vi "Autonomous Independent.vi"() -> ()   [LabVIEW 2016]
doc: "This VI is called when autonomous begins, and will automatically be terminated when autonomous ends. You can carry out timed or sensor driven robot movement independently without needing to return to the caller."
uses:
  Systems/Global 1.vi
  Global 2.vi
  <vilib>/Rock Robotics/Network Tables/NT Read Number.vi
panel:
  out "Present (s)":dbl=3575828146.202245
  out "Time has Elapsed":bool=TRUE
  out "Elapsed Time (s)":dbl=0.5143580436706543
  out "Gyro":dbl=31.8801500557848
  in  "Oscillate effort":dbl=0.25 format="%#_13g"
  out "Auto Mode":dbl=5.0
  in  "Auton_Modes":T1(array[cluster])=[{"Actions"=[{"Effort"=0.55, "Duration"=3.5, "Action"=enum."Vision Correction", "Encoder"=0.0, "Condition"=FALSE}, {"Effort"=0.0, "Duration"=0.0, "Action"=enum."Nothing", "Encoder"=0.0, "Condition"=FALSE}]}, {"Actions"=[{"Effort"=0.0, "Duration"=0.1, "Action"=enum."Drive Encoder Reset", "Encoder"=0.0, "Condition"=FALSE}, {"Effort"=0.0, "Duration"=0.1, "Action"=enum."Gyro Reset", "Encoder"=0.0, "Condition"=FALSE}, {"Effort"=0.4, "Duration"=4.0, "Action"=enum."Drive", "Encoder"=62.0, "Condition"=FALSE}, {"Effort"=0.18, "Duration"=1.0, "Action"=enum."Turn", "Encoder"=-60.0, "Condition"=FALSE}, {"Effort"=0.0, "Duration"=0.1, "Action"=enum."Drive Encoder Reset", "Encoder"=0.0, "Condition"=FALSE}, {"Effort"=0.4, "Duration"=4.0, "Action"=enum."Drive", "Encoder"=65.5, "Condition"=FALSE}, {"Effort"=1.0, "Duration"=0.25, "Action"=enum."Gear0", "Encoder"=0.0, "Condition"=FALSE}, {"Effort"=-0.3, "Duration"=0.1, "Action"=enum."Drive Encoder Reset", "Encoder"=24.0, "Condition"=FALSE}, {"Effort"=-0.4, "Duration"=3.0, "Action"=enum."Drive", "Encoder"=36.0, "Condition"=FALSE}, {"Effort"=0.0, "Duration"=0.0, "Action"=enum."Turn", "Encoder"=31.5, "Condition"=FALSE}, {"Effort"=0.0, "Duration"=0.1, "Action"=enum."Drive Encoder Reset", "Encoder"=0.0, "Condition"=FALSE}, {"Effort"=-0.4, "Duration"=5.0, "Action"=enum."Drive", "Encoder"=70.0, "Condition"=TRUE}]}, {"Actions"=[{"Effort"=0.0, "Duration"=0.1, "Action"=enum."Drive Encoder Reset", "Encoder"=0.0, "Condition"=FALSE}, {"Effort"=0.0, "Duration"=0.1, "Action"=enum."Gyro Reset", "Encoder"=0.0, "Condition"=FALSE}, {"Effort"=0.3, "Duration"=4.0, "Action"=enum."Drive", "Encoder"=75.0, "Condition"=FALSE}, {"Effort"=1.0, "Duration"=1.0, "Action"=enum."Gear0", "Encoder"=0.0, "Condition"=FALSE}, {"Effort"=1.0, "Duration"=0.0, "Action"=enum."Nothing", "Encoder"=0.0, "Condition"=FALSE}, {"Effort"=1.0, "Duration"=0.0, "Action"=enum."Nothing", "Encoder"=0.0, "Condition"=FALSE}, {"Effort"=0.0, "Duration"=0.0, "Action"=enum."Drive Encoder Reset", "Encoder"=0.0, "Condition"=FALSE}, {"Effort"=0.0, "Duration"=0.0, "Action"=enum."Nothing", "Encoder"=0.0, "Condition"=FALSE}, {"Effort"=0.0, "Duration"=0.0, "Action"=enum."Nothing", "Encoder"=0.0, "Condition"=FALSE}, {"Effort"=-0.2, "Duration"=10000.0, "Action"=enum."Drive", "Encoder"=24.0, "Condition"=FALSE}, {"Effort"=0.0, "Duration"=0.0, "Action"=enum."Drive Encoder Reset", "Encoder"=0.0, "Condition"=FALSE}, {"Effort"=-0.4, "Duration"=5.0, "Action"=enum."Nothing", "Encoder"=70.0, "Condition"=FALSE}]}, {"Actions"=[{"Effort"=0.0, "Duration"=0.1, "Action"=enum."Drive Encoder Reset", "Encoder"=6.462, "Condition"=FALSE}, {"Effort"=0.0, "Duration"=0.1, "Action"=enum."Gyro Reset", "Encoder"=0.0, "Condition"=FALSE}, {"Effort"=-0.25, "Duration"=1.0, "Action"=enum."Drive", "Encoder"=6.462, "Condition"=FALSE}, {"Effort"=0.0, "Duration"=0.1, "Action"=enum."Gyro Reset", "Encoder"=0.0, "Condition"=FALSE}, {"Effort"=-0.25, "Duration"=0.0, "Action"=enum."Turn", "Encoder"=0.0, "Condition"=FALSE}, {"Effort"=-0.25, "Duration"=0.0, "Action"=enum."Drive", "Encoder"=7.5, "Condition"=FALSE}, {"Effort"=-1.0, "Duration"=0.0, "Action"=enum."Gear0", "Encoder"=0.0, "Condition"=FALSE}, {"Effort"=0.25, "Duration"=0.0, "Action"=enum."Drive", "Encoder"=3.0, "Condition"=FALSE}]}, {"Actions"=[{"Effort"=0.0, "Duration"=0.1, "Action"=enum."Drive Encoder Reset", "Encoder"=6.462, "Condition"=FALSE}, {"Effort"=0.0, "Duration"=0.1, "Action"=enum."Gyro Reset", "Encoder"=0.0, "Condition"=FALSE}, {"Effort"=-0.25, "Duration"=1.0, "Action"=enum."Drive", "Encoder"=6.462, "Condition"=FALSE}, {"Effort"=0.0, "Duration"=0.1, "Action"=enum."Gyro Reset", "Encoder"=0.0, "Condition"=FALSE}, {"Effort"=-0.25, "Duration"=0.0, "Action"=enum."Turn", "Encoder"=0.0, "Condition"=FALSE}, {"Effort"=-0.25, "Duration"=0.0, "Action"=enum."Drive", "Encoder"=7.5, "Condition"=FALSE}, {"Effort"=-1.0, "Duration"=0.0, "Action"=enum."Gear0", "Encoder"=0.0, "Condition"=FALSE}, {"Effort"=0.25, "Duration"=0.0, "Action"=enum."Drive", "Encoder"=3.0, "Condition"=FALSE}]}, {"Actions"=[{"Effort"=0.0, "Duration"=0.1, "Action"=enum."Drive Encoder Reset", "Encoder"=0.0, "Condition"=FALSE}, {"Effort"=0.0, "Duration"=0.1, "Action"=enum."Gyro Reset", "Encoder"=0.0, "Condition"=FALSE}, {"Effort"=0.4, "Duration"=4.0, "Action"=enum."Drive", "Encoder"=62.0, "Condition"=FALSE}, {"Effort"=0.18, "Duration"=0.1, "Action"=enum."Turn", "Encoder"=60.0, "Condition"=FALSE}, {"Effort"=0.0, "Duration"=0.1, "Action"=enum."Drive Encoder Reset", "Encoder"=0.0, "Condition"=FALSE}, {"Effort"=0.4, "Duration"=4.0, "Action"=enum."Drive", "Encoder"=65.5, "Condition"=FALSE}, {"Effort"=1.0, "Duration"=0.25, "Action"=enum."Gear0", "Encoder"=0.0, "Condition"=FALSE}, {"Effort"=0.0, "Duration"=0.1, "Action"=enum."Drive Encoder Reset", "Encoder"=3.0, "Condition"=FALSE}, {"Effort"=-0.4, "Duration"=3.0, "Action"=enum."Drive", "Encoder"=36.0, "Condition"=FALSE}, {"Effort"=0.0, "Duration"=0.0, "Action"=enum."Turn", "Encoder"=31.5, "Condition"=FALSE}, {"Effort"=0.0, "Duration"=0.1, "Action"=enum."Drive Encoder Reset", "Encoder"=0.0, "Condition"=FALSE}, {"Effort"=-0.4, "Duration"=5.0, "Action"=enum."Drive", "Encoder"=70.0, "Condition"=TRUE}]}, {"Actions"=[{"Effort"=0.0, "Duration"=0.1, "Action"=enum."Nothing", "Encoder"=0.0, "Condition"=FALSE}, {"Effort"=0.0, "Duration"=0.1, "Action"=enum."Gyro Reset", "Encoder"=0.0, "Condition"=FALSE}, {"Effort"=0.25, "Duration"=5.0, "Action"=enum."Drive", "Encoder"=60000.0, "Condition"=TRUE}, {"Effort"=0.75, "Duration"=1.0, "Action"=enum."Nothing", "Encoder"=0.0, "Condition"=FALSE}, {"Effort"=0.0, "Duration"=1.0, "Action"=enum."Nothing", "Encoder"=0.0, "Condition"=FALSE}, {"Effort"=0.0, "Duration"=0.0, "Action"=enum."Nothing", "Encoder"=0.0, "Condition"=FALSE}]}, {"Actions"=[{"Effort"=0.0, "Duration"=0.1, "Action"=enum."Drive Encoder Reset", "Encoder"=0.0, "Condition"=FALSE}, {"Effort"=0.0, "Duration"=0.1, "Action"=enum."Gyro Reset", "Encoder"=0.0, "Condition"=FALSE}, {"Effort"=0.3, "Duration"=0.0, "Action"=enum."Drive", "Encoder"=24.0, "Condition"=FALSE}, {"Effort"=0.3, "Duration"=3.0, "Action"=enum."Nothing", "Encoder"=0.0, "Condition"=FALSE}, {"Effort"=0.3, "Duration"=2.0, "Action"=enum."Vision Correction", "Encoder"=30.0, "Condition"=FALSE}, {"Effort"=0.2, "Duration"=1.0, "Action"=enum."Drive", "Encoder"=18.5, "Condition"=TRUE}, {"Effort"=1.0, "Duration"=0.0, "Action"=enum."Gear0", "Encoder"=0.0, "Condition"=FALSE}, {"Effort"=-0.2, "Duration"=1.3, "Action"=enum."Drive", "Encoder"=30.0, "Condition"=TRUE}, {"Effort"=0.0, "Duration"=3.0, "Action"=enum."Nothing", "Encoder"=0.0, "Condition"=FALSE}, {"Effort"=0.03, "Duration"=0.0, "Action"=enum."Turn", "Encoder"=0.0, "Condition"=FALSE}, {"Effort"=0.0, "Duration"=0.0, "Action"=enum."Drive", "Encoder"=0.0, "Condition"=FALSE}]}, {"Actions"=[{"Effort"=0.0, "Duration"=0.0, "Action"=enum."Nothing", "Encoder"=0.0, "Condition"=FALSE}]}, {"Actions"=[{"Effort"=0.0, "Duration"=2.5, "Action"=enum."Shoot", "Encoder"=0.0, "Condition"=FALSE}, {"Effort"=0.0, "Duration"=5.0, "Action"=enum."Index", "Encoder"=0.0, "Condition"=FALSE}, {"Effort"=0.25, "Duration"=3.5, "Action"=enum."Nothing", "Encoder"=88.0, "Condition"=FALSE}, {"Effort"=1.0, "Duration"=1.0, "Action"=enum."Nothing", "Encoder"=0.0, "Condition"=FALSE}, {"Effort"=1.0, "Duration"=1.0, "Action"=enum."Nothing", "Encoder"=0.0, "Condition"=FALSE}, {"Effort"=1.0, "Duration"=0.5, "Action"=enum."Nothing", "Encoder"=0.0, "Condition"=FALSE}, {"Effort"=0.0, "Duration"=0.0, "Action"=enum."Nothing", "Encoder"=0.0, "Condition"=FALSE}, {"Effort"=-0.25, "Duration"=0.0, "Action"=enum."Nothing", "Encoder"=3.0, "Condition"=FALSE}, {"Effort"=0.0, "Duration"=0.0, "Action"=enum."Nothing", "Encoder"=0.0, "Condition"=FALSE}, {"Effort"=0.25, "Duration"=0.0, "Action"=enum."Nothing", "Encoder"=24.0, "Condition"=FALSE}, {"Effort"=0.0, "Duration"=0.0, "Action"=enum."Nothing", "Encoder"=0.0, "Condition"=FALSE}, {"Effort"=-0.25, "Duration"=0.0, "Action"=enum."Nothing", "Encoder"=12.0, "Condition"=FALSE}]}, {"Actions"=[{"Effort"=0.0, "Duration"=0.1, "Action"=enum."Drive Encoder Reset", "Encoder"=0.0, "Condition"=FALSE}, {"Effort"=0.0, "Duration"=1.0, "Action"=enum."Gyro Reset", "Encoder"=0.0, "Condition"=FALSE}, {"Effort"=0.3, "Duration"=1.4, "Action"=enum."Drive", "Encoder"=88.0, "Condition"=FALSE}, {"Effort"=0.3, "Duration"=3.0, "Action"=enum."Turn", "Encoder"=2.0, "Condition"=FALSE}, {"Effort"=1.0, "Duration"=1.0, "Action"=enum."Nothing", "Encoder"=0.0, "Condition"=FALSE}, {"Effort"=1.0, "Duration"=1.0, "Action"=enum."Nothing", "Encoder"=0.0, "Condition"=FALSE}, {"Effort"=0.0, "Duration"=0.0, "Action"=enum."Nothing", "Encoder"=0.0, "Condition"=FALSE}, {"Effort"=-0.25, "Duration"=0.0, "Action"=enum."Nothing", "Encoder"=3.0, "Condition"=FALSE}, {"Effort"=0.0, "Duration"=0.0, "Action"=enum."Nothing", "Encoder"=0.0, "Condition"=FALSE}, {"Effort"=0.25, "Duration"=0.0, "Action"=enum."Nothing", "Encoder"=24.0, "Condition"=FALSE}, {"Effort"=0.0, "Duration"=0.0, "Action"=enum."Nothing", "Encoder"=0.0, "Condition"=FALSE}, {"Effort"=-0.25, "Duration"=0.0, "Action"=enum."Nothing", "Encoder"=12.0, "Condition"=FALSE}]}, {"Actions"=[{"Effort"=0.0, "Duration"=1.0, "Action"=enum."Drive Encoder Reset", "Encoder"=0.0, "Condition"=FALSE}, {"Effort"=0.0, "Duration"=1.0, "Action"=enum."Shoot", "Encoder"=0.0, "Condition"=FALSE}, {"Effort"=0.25, "Duration"=5.0, "Action"=enum."Index", "Encoder"=88.0, "Condition"=FALSE}, {"Effort"=1.0, "Duration"=1.0, "Action"=enum."Nothing", "Encoder"=0.0, "Condition"=FALSE}, {"Effort"=1.0, "Duration"=1.0, "Action"=enum."Nothing", "Encoder"=0.0, "Condition"=FALSE}, {"Effort"=1.0, "Duration"=0.5, "Action"=enum."Nothing", "Encoder"=0.0, "Condition"=FALSE}, {"Effort"=0.0, "Duration"=0.0, "Action"=enum."Nothing", "Encoder"=0.0, "Condition"=FALSE}, {"Effort"=-0.25, "Duration"=0.0, "Action"=enum."Nothing", "Encoder"=3.0, "Condition"=FALSE}, {"Effort"=0.0, "Duration"=0.0, "Action"=enum."Nothing", "Encoder"=0.0, "Condition"=FALSE}, {"Effort"=0.25, "Duration"=0.0, "Action"=enum."Nothing", "Encoder"=24.0, "Condition"=FALSE}, {"Effort"=0.0, "Duration"=0.0, "Action"=enum."Nothing", "Encoder"=0.0, "Condition"=FALSE}, {"Effort"=-0.25, "Duration"=0.0, "Action"=enum."Nothing", "Encoder"=12.0, "Condition"=FALSE}]}, {"Actions"=[{"Effort"=0.0, "Duration"=0.1, "Action"=enum."Drive Encoder Reset", "Encoder"=0.0, "Condition"=FALSE}, {"Effort"=0.0, "Duration"=1.0, "Action"=enum."Gyro Reset", "Encoder"=0.0, "Condition"=FALSE}, {"Effort"=0.3, "Duration"=1.4, "Action"=enum."Drive", "Encoder"=88.0, "Condition"=FALSE}, {"Effort"=0.3, "Duration"=4.0, "Action"=enum."Turn", "Encoder"=0.0, "Condition"=FALSE}, {"Effort"=1.0, "Duration"=1.0, "Action"=enum."Nothing", "Encoder"=0.0, "Condition"=FALSE}, {"Effort"=1.0, "Duration"=0.5, "Action"=enum."Nothing", "Encoder"=0.0, "Condition"=FALSE}, {"Effort"=0.0, "Duration"=0.0, "Action"=enum."Nothing", "Encoder"=0.0, "Condition"=FALSE}, {"Effort"=0.3, "Duration"=0.5, "Action"=enum."Nothing", "Encoder"=24.0, "Condition"=TRUE}, {"Effort"=0.0, "Duration"=0.0, "Action"=enum."Nothing", "Encoder"=0.0, "Condition"=FALSE}, {"Effort"=-0.2, "Duration"=2.0, "Action"=enum."Nothing", "Encoder"=24.0, "Condition"=TRUE}, {"Effort"=0.0, "Duration"=0.0, "Action"=enum."Nothing", "Encoder"=0.0, "Condition"=FALSE}, {"Effort"=-0.25, "Duration"=0.0, "Action"=enum."Nothing", "Encoder"=12.0, "Condition"=FALSE}]}]
  # "Nothing"
  # "Boiler Right Right side gear"
  # "Middle Gear"
  # "Boiler Right Left Side Gear"
  # "Boiler Left RightSide Gear"
  # "Boiler Left Left Side Gear"
  # "Drive"
  # "Vision Correction"
  # "Hopper"
  # "10 ball"
  # "Farside"
  # "Boilerside-10 ball"
  # "Auto 5"
  # "Auto 6"
  # "Auto 6"
  # "Auto 7"
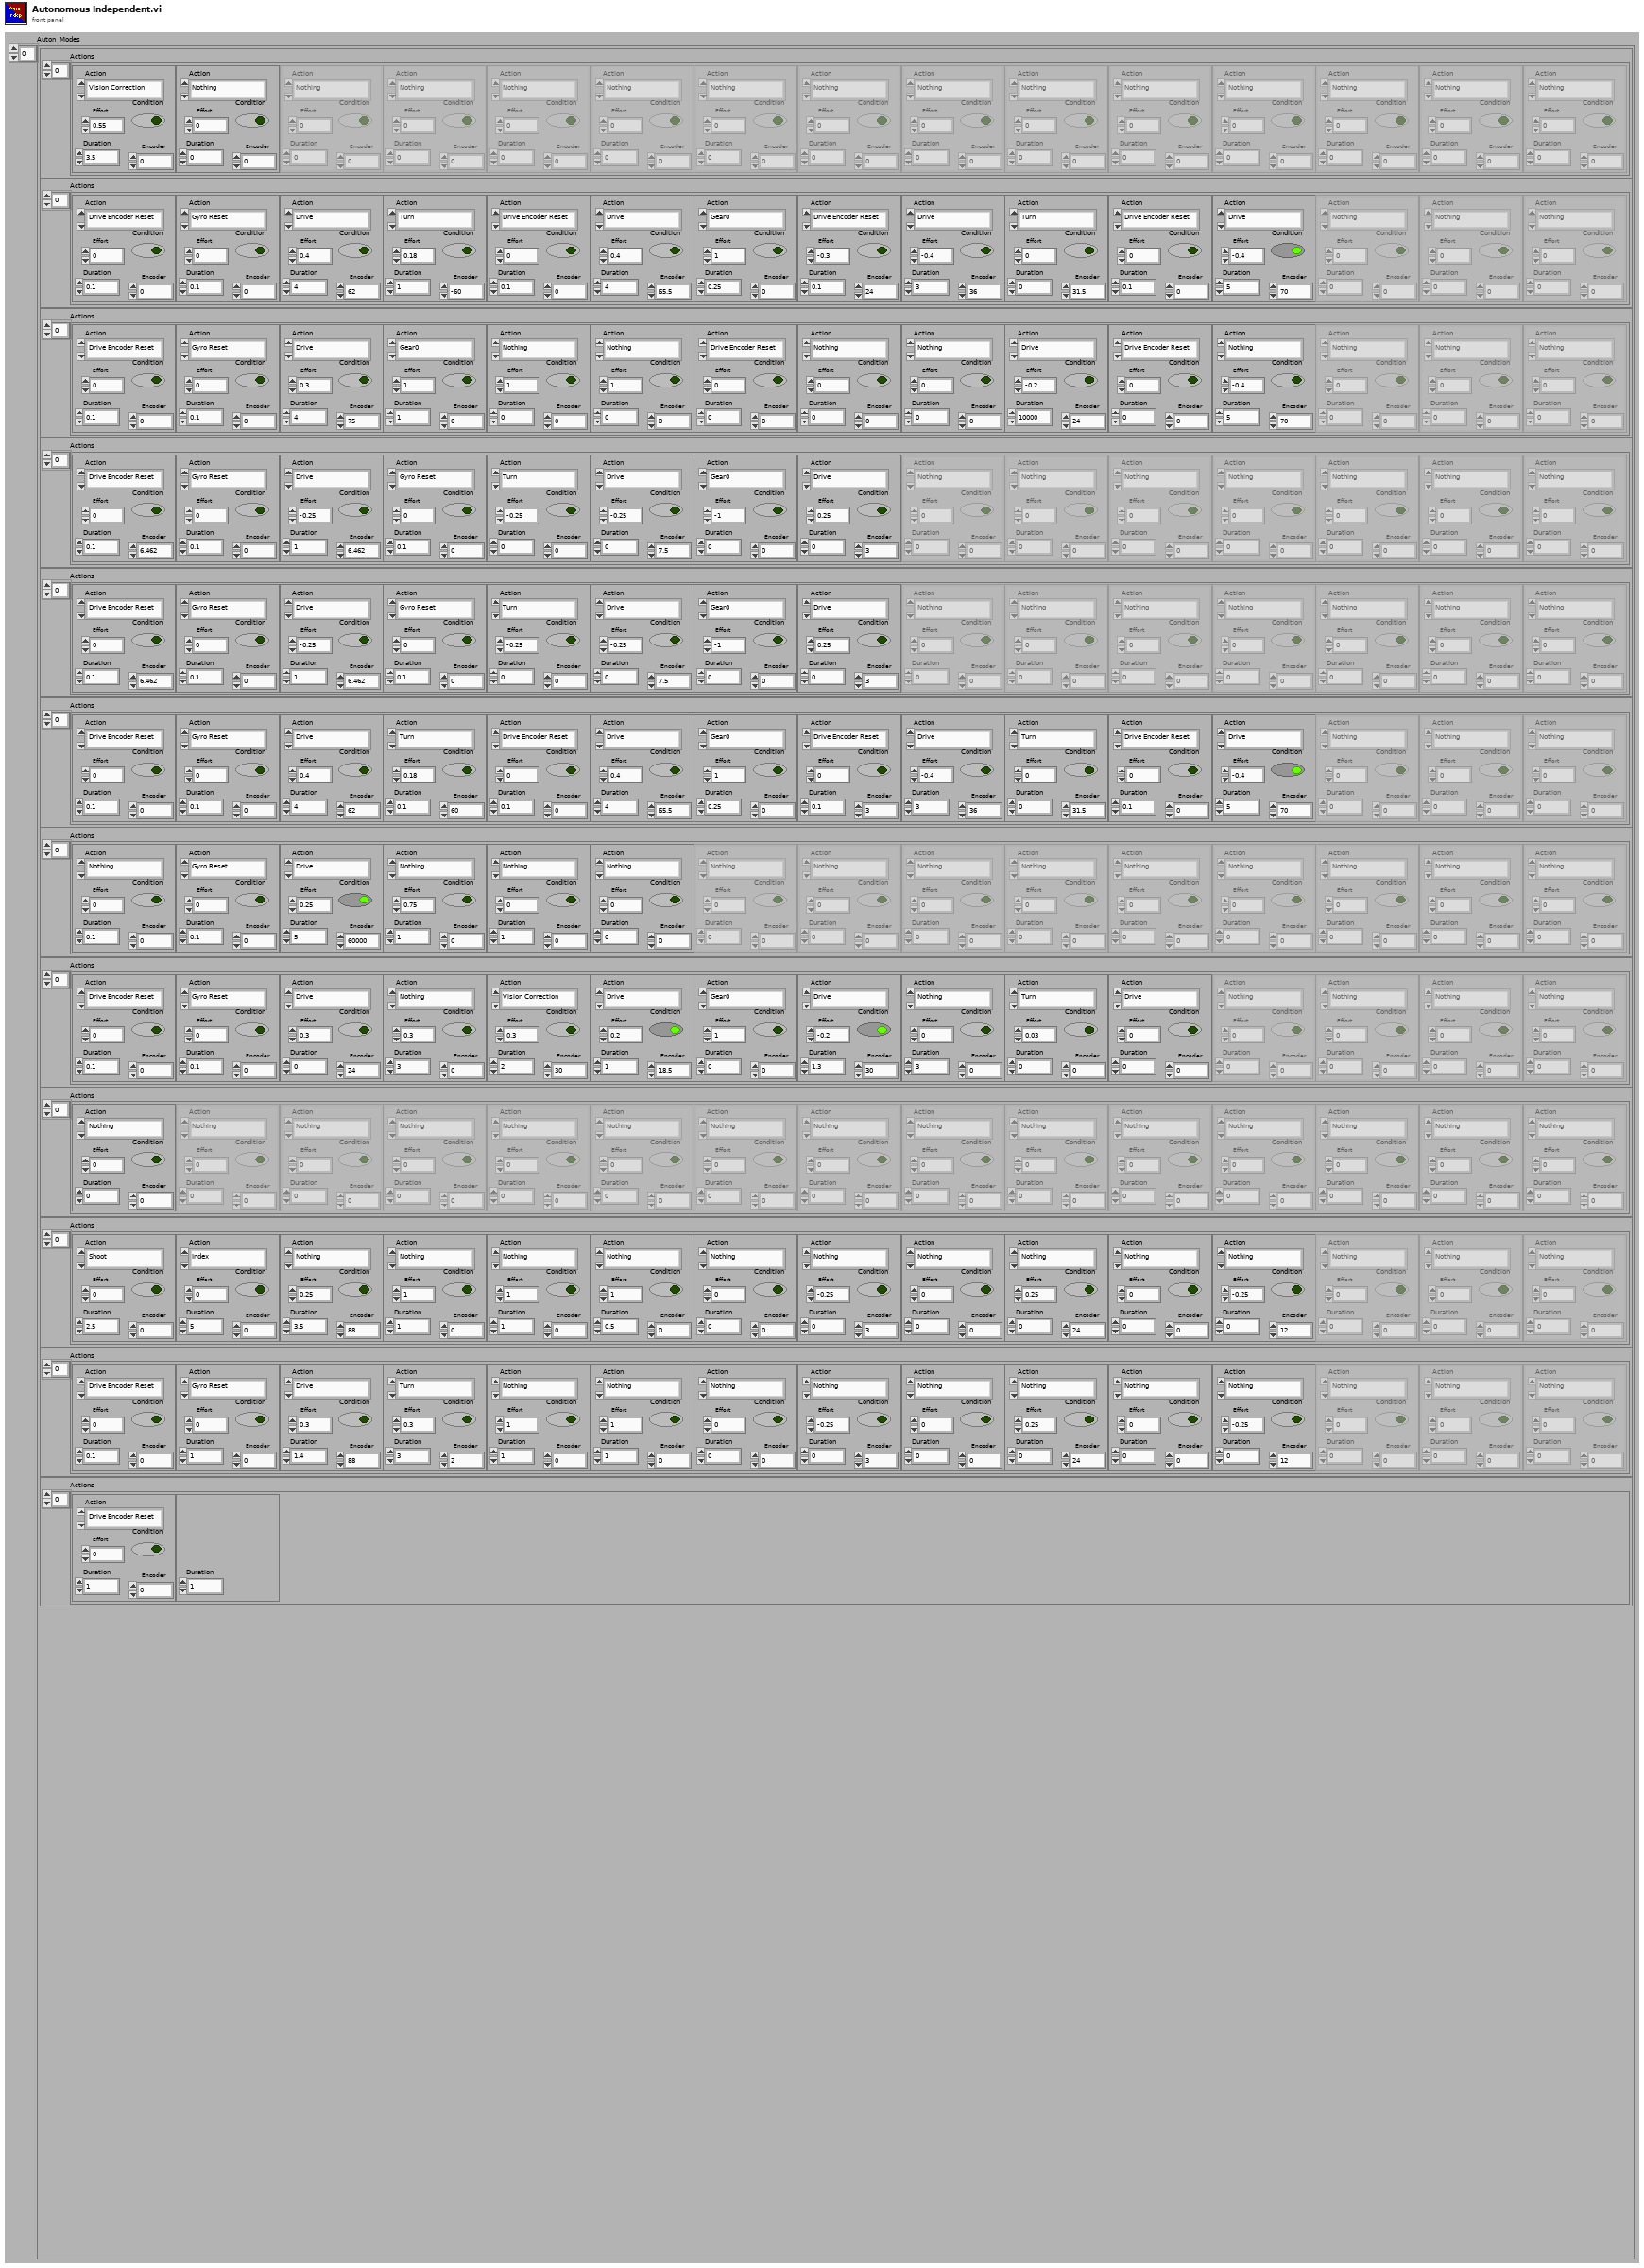
[diagram p1: front panel]
types:
  T1 = cluster{"Actions":cluster{"Effort":dbl, "Duration":dbl, "Action":enum16{"Nothing", "Drive", "Vision Correction", "Turn", "Gear0", "Gear1", "Climb", "Intake", "Index", "Shoot", "Test", "Drive Encoder Reset", "Gyro Reset"}, "Encoder":dbl, "Condition":bool}[]}[]
  T2 = cluster{"Actions":cluster{"Effort":dbl, "Duration":dbl, "Action":enum16{"Nothing", "Drive", "Vision Correction", "Turn", "Gear0", "Gear1", "Climb", "Intake", "Index", "Shoot", "Test", "Drive Encoder Reset", "Gyro Reset"}, "Encoder":dbl, "Condition":bool}[]}
  T3 = cluster{"Effort":dbl, "Duration":dbl, "Action":enum16{"Nothing", "Drive", "Vision Correction", "Turn", "Gear0", "Gear1", "Climb", "Intake", "Index", "Shoot", "Test", "Drive Encoder Reset", "Gyro Reset"}, "Encoder":dbl, "Condition":bool}[]
  T4 = enum16{"Nothing", "Drive", "Vision Correction", "Turn", "Gear0", "Gear1", "Climb", "Intake", "Index", "Shoot", "Test", "Drive Encoder Reset", "Gyro Reset"}
  T5 = typedef "WPI_MotorControlDeviceRef.ctl" = cluster{"DeviceStatus":errorcluster, "Type":T6, "PWM":cluster{"PWM Channel":T7, "DeadBand":T8}, "CAN":cluster{"Device Number":u8, "SetOutput VI Ref":variant, "GetOutput VI Ref":variant, "Enable VI Ref":variant, "Disable VI Ref":variant, "Data":variant}, "Invert":bool}
  T6 = typedef "WPI_MotorControlType.ctl" = enum16{"PWM", "CAN"}
  T7 = typedef "FPGA_DIOPWMChannel.ctl" = enum8{"PWM 0", "PWM 1", "PWM 2", "PWM 3", "PWM 4", "PWM 5", "PWM 6", "PWM 7", "PWM 8", "PWM 9", "PWM MXP 0", "PWM MXP 1", "PWM MXP 2", "PWM MXP 3", "PWM MXP 4", "PWM MXP 5", "PWM MXP 6", "PWM MXP 7", "PWM MXP 8", "PWM MXP 9", "Invalid"}
  T8 = typedef "WPI_PWMDeadband.ctl" = cluster{"Name":string, "maxPositivePwm":i32, "minPositivePwm":i32, "centerPwm":i32, "maxNegativePwm":i32, "minNegativePwm":i32, "angularRange":u16}
  T9 = typedef "WPI_CANTalonSRX_GlobalStatus.ctl" = cluster{"Applied Throttle":dbl, "Module Enabled":bool, "CAN Error":errorcluster, "Closed Loop Error":dbl, "Forward Limit Switch Closed":bool, "Reverse Limit Switch Closed":bool, "Sensor Position":dbl, "Sensor Velocity":dbl, "Current":dbl, "Sticky Fault - Over Temp":bool, "Sticky Fault - Under Voltage":bool, "Sticky Fault - Forward Limit":bool, "Sticky Fault - Reverse Limit":bool, "Sticky Fault - Forward Soft Limit":bool, "Sticky Fault - Reverse Soft Limit":bool, "Brake is Enabled":bool, "Encoder Position":dbl, "Encoder Velocity":dbl, "Encoder Index Count":dbl, "Encoder A Pin State":bool, "Encoder B Pin State":bool, "Encoder Index Pin State":bool, "Analog In":dbl, "Analog In Velocity":dbl, "Temperature (C)":dbl, "Battery Voltage":dbl, "Control 5 Is Supported":bool, "Current Profile Slot Select":dbl, "Pos Div 8":bool, "Vel Div 4":bool, "Pulse Width Position":i32, "Pulse Width Velocity":i32, "Pulse Width Rise To Rise (us)":i32, "Pulse Width Rise To Fall (us)":i32, "Mot Prof Active Is Under Run":bool, "Mot Prof Active Has Under Run":bool, "Mot Prof Active Is Last":bool, "Mot Prof Active Velocity Only":bool, "Mot Prof Active Is Valid":bool, "Mot Prof Buffer Is Full":bool, "Mot Prof Active Profile Slot Select":i32, "Mot Prof NextID":i32, "Mot Prof Count":i32, "Mot Prof Active Velocity":dbl, "Mot Prof Active Position":dbl, "Mot Prof Output Enable":i32}
  T10 = typedef "WPI_GyroDevRef.ctl" = cluster{"DevStatus":errorcluster, "Analog Channel":T11, "Offset":dbl, "Gain (VoltsPerDegree/Second)":dbl, "Gyro Type":enum16{"Analog", "XRS450"}, "Handle":i32, "SPI Bus":T12, "Device Found":bool, "Sample Rate":dbl, "Calibrate On Open":bool}
  T11 = typedef "FPGA_AIChannel.ctl" = enum8{"AI 0", "AI 1", "AI 2", "AI 3", "AI MXP 0", "AI MXP 1", "AI MXP 2", "AI MXP 3", "Invalid"}
  T12 = typedef "spi_bus.ctl" = enum16{"SPI On-Board, CS0", "SPI On-Board, CS1", "SPI On-Board, CS2", "SPI On-Board, CS3", "SPI MXP", "Invalid"}
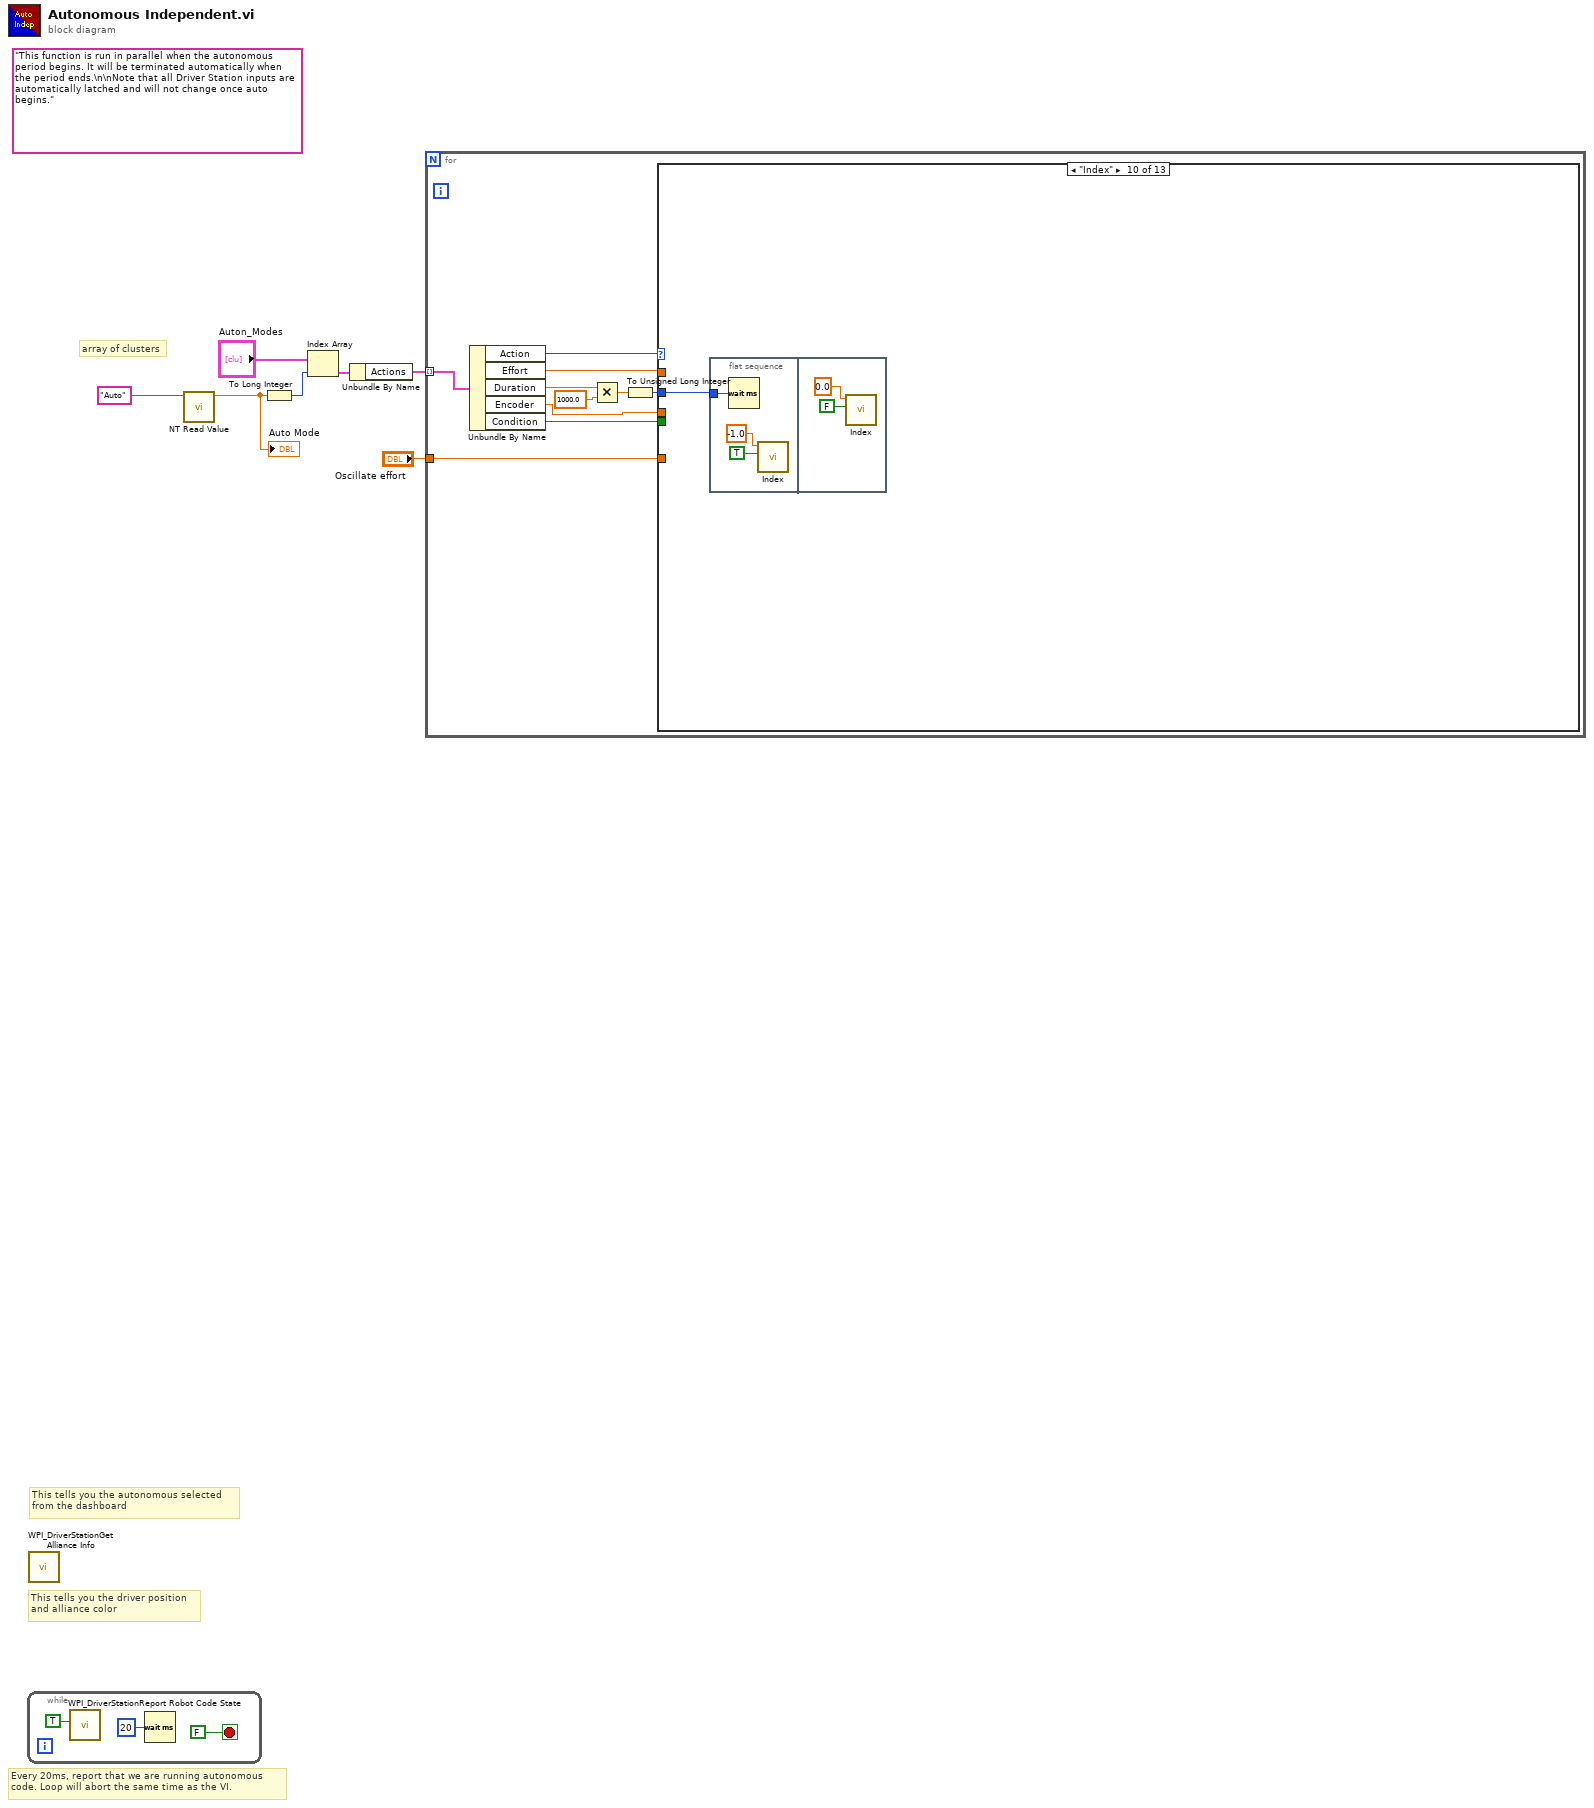
[diagram p0: block diagram]
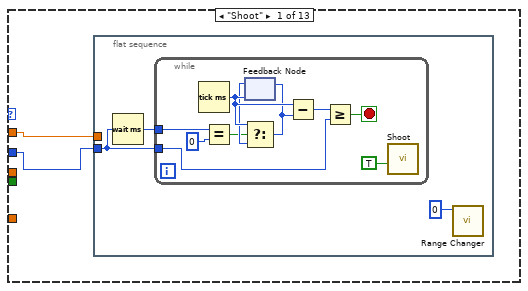
[diagram p2: hidden frame]
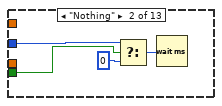
[diagram p3: hidden frame]
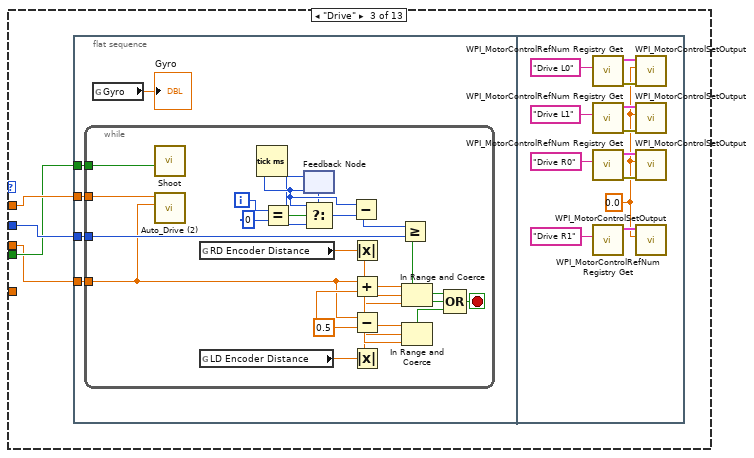
[diagram p4: hidden frame]
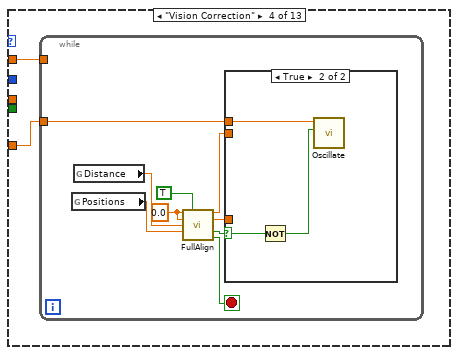
[diagram p5: hidden frame]
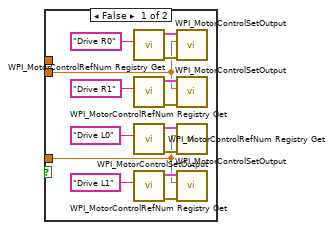
[diagram p6: hidden frame]
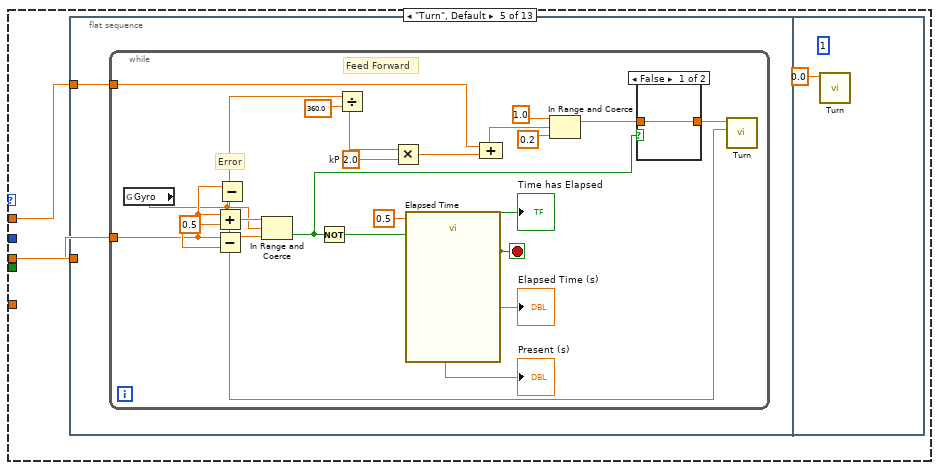
[diagram p7: hidden frame]
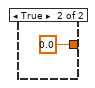
[diagram p8: hidden frame]
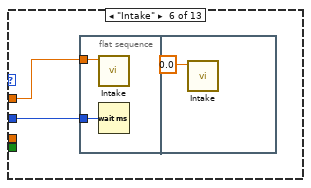
[diagram p9: hidden frame]
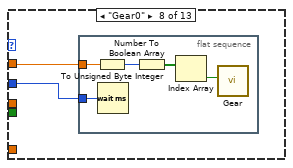
[diagram p11: hidden frame]
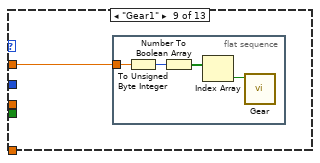
[diagram p12: hidden frame]
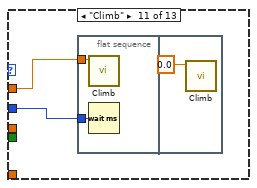
[diagram p13: hidden frame]
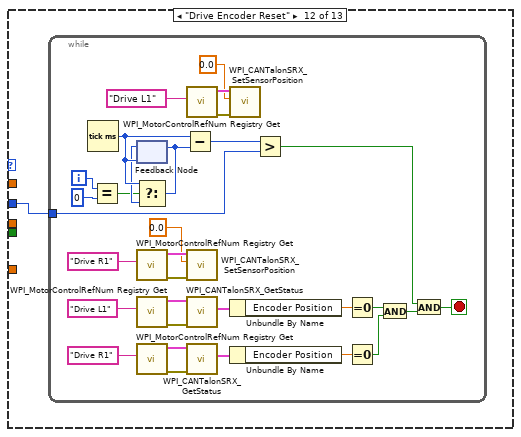
[diagram p14: hidden frame]
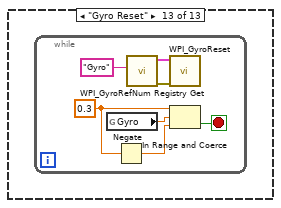
[diagram p15: hidden frame]
diagram:
  (unwired) "This function is run in parallel when the autonomous period begins. It will be terminated automatically when the period ends.\n\nNote that all Driver Station inputs are automatically latched and will not change once auto begins."
  # "This tells you the autonomous selected\nfrom the dashboard"
  # "array of clusters"
  # "Every 20ms, report that we are running autonomous\ncode. Loop will abort the same time as the VI."
  # "This tells you the driver position\nand alliance color"
  n1 = while {
    stop <- FALSE stop-if-true
    n2 = call <vilib>:"WPI_DriverStationReport Robot Code State.vi"("Autonomous"=TRUE) -> ()  [unwired: 10 in, 1 out]
    n3 = Wait (ms)(milliseconds to wait=u32 20) -> ()  [unwired: 1 out]
  }
  n4 = call <vilib>:"WPI_DriverStationGet Alliance Info.vi"() -> ()  [unwired: 12 out]
  n5 = call-poly <vilib>:"NT Read Value.vi"("Name"="Auto") -> ("Numeric"=w2:dbl)  [unwired: 9 in, 1 out]
  "Auto Mode" <- w2
  n6 = To Long Integer(number=w2) -> (32bit integer=w4:i32)
  n7 = Index Array(array="Auton_Modes", index=w4) -> (element=w6:T2)
  n8 = Unbundle By Name(w6) -> ("Actions"=w7:T3)
  n9 = for {
    tunnel: w7 -> [w20] mode=indexing
    tunnel: "Oscillate effort" -> [w12]
    n10 = Unbundle By Name(w20) -> ("Action"=w11:T4, "Effort"=w19:dbl, "Duration"=w18:dbl, "Encoder"=w13:dbl, "Condition"=w15:bool)
    n11 = Multiply(x=w18, y=1000.0) -> (x*y=w17:dbl)
    n12 = To Unsigned Long Integer(number=w17) -> (unsigned 32bit integer=w16:u32)
    n13 = case shown="\"Index\"" w11 {
      tunnel: w19 -> [w22 _ w43 w84 w112 w141 _ w146 w152 _ w164 _ _]
      tunnel: w16 -> [w21 w38 w42 _ _ w140 _ w145 _ w157 w163 w168 _]
      tunnel: w15 -> [_ w39 w41 _ _ _ _ _ _ _ _ _ _]
      tunnel: w13 -> [_ _ w40 _ w111 _ _ _ _ _ _ _ _]
      tunnel: w12 -> [_ _ _ w83 _ _ _ _ _ _ _ _ _]
      frame "Shoot" {
        n14 = flat-sequence {
          tunnel: w22 -> [_]
          tunnel: w21 -> [w23]
          frame #0 {
            n15 = Wait (ms)(milliseconds to wait=w23) -> (millisecond timer value=w24:u32)
            n16 = while {
              tunnel: w24 -> [w27]
              tunnel: w23 -> [w26]
              stop <- w28 stop-if-true
              n17 = Tick Count (ms)() -> (millisecond timer value=w34:u32)
              n18 = Equal?(x=w27, y=0) -> (x = y?=w32:bool)
              n19 = feedback #1(w34) -> (w33:u32)
              n20 = Select(t=w34, s=w32, f=w33) -> (s? t:f=w30:u32)
              n21 = feedback-in #1(w30) -> ()
              n22 = Subtract(x=w34, y=w30) -> (x-y=w29:u32)
              n23 = Greater Or Equal?(x=w29, y=w26) -> (x >= y?=w28:bool)
              n24 = call "Shoot.vi"("Shoot"=TRUE) -> ()  [unwired: 10 in]
            }
            n25 = call "Range Changer.vi"("POV"=i16 0) -> ()  [unwired: 10 in, 1 out]
          }
        }
      }
      frame "Nothing" {
        n26 = Select(t=w38, s=w39, f=u32 0) -> (s? t:f=w36:u32)
        n27 = Wait (ms)(milliseconds to wait=w36) -> ()  [unwired: 1 out]
      }
      frame "Drive" {
        n28 = flat-sequence {
          tunnel: w43 -> [w48]
          tunnel: w42 -> [w44]
          tunnel: w41 -> [w46]
          tunnel: w40 -> [w47]
          frame #0 {
            n29 = while {
              tunnel: w48 -> [w70]
              tunnel: w47 -> [w49]
              tunnel: w46 -> [w53]
              tunnel: w44 -> [w63]
              i -> [w62]
              stop <- w56 stop-if-true
              w61 = 0.5 ("Range")
              n30 = call "Shoot.vi"("Shoot"=w53) -> ()  [unwired: 10 in]
              n31 = call "Auto_Drive (2).vi"("Target"=w49, "Drive Effort"=w70) -> ()  [unwired: 10 in]
              n32 = global read "Global 2.vi" "RD Encoder Distance"() -> (w58:dbl)
              n33 = global read "Global 2.vi" "LD Encoder Distance"() -> (w57:dbl)
              n34 = Tick Count (ms)() -> (millisecond timer value=w69:u32)
              n35 = Equal?(x=w62, y=0) -> (x = y?=w67:bool)
              n36 = feedback #2(w69) -> (w68:u32)
              n37 = Select(t=w69, s=w67, f=w68) -> (s? t:f=w65:u32)
              n38 = feedback-in #2(w65) -> ()
              n39 = Subtract(x=w69, y=w65) -> (x-y=w64:u32)
              n40 = Absolute Value(x=w58) -> (abs(x)=w55:dbl)
              n41 = Add(x=w49, y=w61) -> (x+y=w60:dbl)
              n42 = Subtract(x=w49, y=w61) -> (x-y=w59:dbl)
              n43 = Absolute Value(x=w57) -> (abs(x)=w54:dbl)
              n44 = Greater Or Equal?(x=w64, y=w63) -> (x >= y?=w50:bool)
              n45 = In Range and Coerce(upper limit=w60, x=w55, lower limit=w59) -> (In Range?=w51:bool)  [unwired: 1 out]
              n46 = In Range and Coerce(upper limit=w60, x=w54, lower limit=w59) -> (In Range?=w52:bool)  [unwired: 1 out]
              n47 = Compound Arithmetic op=OR(w50, w51, w52) -> (w56:bool)
            }
            n48 = global read "Global 2.vi" "Gyro"() -> (→"Gyro":dbl)
          }
          frame #1 {
            w71 = 0.0 ("Drive L")
            n49 = call <vilib>:"WPI_MotorControlRefNum Registry Get.vi"("refnum name"="Drive L0") -> ("error out"=w77:errorcluster, "MotorControlDevRef"=w78:T5)  [unwired: 9 in]
            n50 = call <vilib>:"WPI_MotorControlRefNum Registry Get.vi"("refnum name"="Drive L1") -> ("error out"=w81:errorcluster, "MotorControlDevRef"=w80:T5)  [unwired: 9 in]
            n51 = call <vilib>:"WPI_MotorControlRefNum Registry Get.vi"("refnum name"="Drive R0") -> ("error out"=w76:errorcluster, "MotorControlDevRef"=w72:T5)  [unwired: 9 in]
            n52 = call <vilib>:"WPI_MotorControlRefNum Registry Get.vi"("refnum name"="Drive R1") -> ("MotorControlDevRef"=w74:T5)  [unwired: 9 in, 1 out]
            n53 = call <vilib>:"WPI_MotorControlSetOutput.vi"("error in (no error)"=w77, "Output"=w71, "MotorControlDevRef"=w78) -> ()  [unwired: 6 in, 3 out]
            n54 = call <vilib>:"WPI_MotorControlSetOutput.vi"("error in (no error)"=w81, "Output"=w71, "MotorControlDevRef"=w80) -> ()  [unwired: 6 in, 3 out]
            n55 = call <vilib>:"WPI_MotorControlSetOutput.vi"("error in (no error)"=w76, "Output"=w71, "MotorControlDevRef"=w72) -> ()  [unwired: 6 in, 3 out]
            n56 = call <vilib>:"WPI_MotorControlSetOutput.vi"("Output"=w71, "MotorControlDevRef"=w74) -> ()  [unwired: 7 in, 3 out]
          }
        }
      }
      frame "Vision Correction" {
        n57 = while {
          tunnel: w84 -> [_]
          tunnel: w83 -> [w87]
          stop <- w88 stop-if-true
          w91 = 0.0
          n58 = global read "Global 1.vi" "Positions"() -> (w89:dbl)
          n59 = global read "Global 1.vi" "Distance"() -> (w90:dbl)
          n60 = call "FullAlign.vi"("Joystick 0"=w91, "Button"=TRUE, "Joystick 1"=w91, "Distance"=w90, "Angle"=w89) -> ("Right Motor"=w93:dbl, "Left Motor"=w92:dbl, "Not In Sight?"=w85:bool, "In Range?"=w88:bool)  [unwired: 7 in]
          n61 = case shown="True" w85 {
            selector: w85 -> [_ w110]
            tunnel: w93 -> [w95 _]
            tunnel: w92 -> [w94 _]
            tunnel: w87 -> [_ w108]
            frame False {
              n62 = call <vilib>:"WPI_MotorControlRefNum Registry Get.vi"("refnum name"="Drive R0") -> ("error out"=w101:errorcluster, "MotorControlDevRef"=w97:T5)  [unwired: 9 in]
              n63 = call <vilib>:"WPI_MotorControlRefNum Registry Get.vi"("refnum name"="Drive R1") -> ("error out"=w96:errorcluster, "MotorControlDevRef"=w99:T5)  [unwired: 9 in]
              n64 = call <vilib>:"WPI_MotorControlRefNum Registry Get.vi"("refnum name"="Drive L0") -> ("error out"=w102:errorcluster, "MotorControlDevRef"=w103:T5)  [unwired: 9 in]
              n65 = call <vilib>:"WPI_MotorControlRefNum Registry Get.vi"("refnum name"="Drive L1") -> ("error out"=w106:errorcluster, "MotorControlDevRef"=w105:T5)  [unwired: 9 in]
              n66 = call <vilib>:"WPI_MotorControlSetOutput.vi"("error in (no error)"=w101, "Output"=w95, "MotorControlDevRef"=w97) -> ()  [unwired: 6 in, 3 out]
              n67 = call <vilib>:"WPI_MotorControlSetOutput.vi"("error in (no error)"=w96, "Output"=w95, "MotorControlDevRef"=w99) -> ()  [unwired: 6 in, 3 out]
              n68 = call <vilib>:"WPI_MotorControlSetOutput.vi"("error in (no error)"=w102, "Output"=w94, "MotorControlDevRef"=w103) -> ()  [unwired: 6 in, 3 out]
              n69 = call <vilib>:"WPI_MotorControlSetOutput.vi"("error in (no error)"=w106, "Output"=w94, "MotorControlDevRef"=w105) -> ()  [unwired: 6 in, 3 out]
            }
            frame True {
              n70 = Not(x=w110) -> (.not. x?=w109:bool)
              n71 = call "Oscillate.vi"("Target In Sight?"=w109, "Effort"=w108) -> ()  [unwired: 10 in]
            }
          }
        }
      }
      frame "Turn", Default {
        n72 = flat-sequence {
          tunnel: w112 -> [w114]
          tunnel: w111 -> [w113]
          frame #0 {
            n73 = while {
              tunnel: w114 -> [w123]
              tunnel: w113 -> [w126]
              stop <- w129 stop-if-true
              w124 = 2.0  # kP
              w136 = 0.5
              # "Feed Forward"
              # "Error"
              n74 = global read "Global 2.vi" "Gyro"() -> (w125:dbl)
              n75 = Add(x=w126, y=w136) -> (x+y=w135:dbl)
              n76 = Subtract(x=w126, y=w136) -> (x-y=w134:dbl)
              n77 = Subtract(x=w126, y=w125) -> (x-y=w115:dbl)
              n78 = In Range and Coerce(upper limit=w135, x=w125, lower limit=w134) -> (In Range?=w128:bool)  [unwired: 1 out]
              n79 = Not(x=w128) -> (.not. x?=w130:bool)
              n80 = Divide(x=w115, y=360.0 ("x-y")) -> (x/y=w120:dbl)
              n81 = Multiply(x=w120, y=w124) -> (x*y=w122:dbl)
              n82 = call "Elapsed Time"("Time Target (s)"=0.5, "Reset"=w130) -> ("Present (s)"=→"Present (s)":dbl, "Elapsed Time (s)"=→"Elapsed Time (s)":dbl, "Time has Elapsed"=w129:bool)  [unwired: 10 in, 5 out]
              "Time has Elapsed" <- w129
              n83 = Compound Arithmetic op=ADD(w123, w122) -> (w121:dbl)
              n84 = In Range and Coerce(upper limit=1.0, x=w121, lower limit=0.2) -> (coerced(x)=w118:dbl)  [unwired: 1 out]
              n85 = case shown="False" w128 {
                tunnel: [w137 0.0] -> w127
                tunnel: w118 -> [w137 _]
                frame False {
                }
                frame True {
                }
              }
              n86 = call "Turn.vi"("Gyro"=w115, "Effort"=w127) -> ()  [unwired: 10 in]
            }
          }
          frame #1 {
            (unwired) 1 ("mode")
            n87 = call "Turn.vi"("Effort"=0.0) -> ()  [unwired: 11 in]
          }
        }
      }
      frame "Intake" {
        n88 = flat-sequence {
          tunnel: w141 -> [w143]
          tunnel: w140 -> [w142]
          frame #0 {
            n89 = call "Intake.vi"("Effort"=w143) -> ()  [unwired: 11 in]
            n90 = Wait (ms)(milliseconds to wait=w142) -> ()  [unwired: 1 out]
          }
          frame #1 {
            n91 = call "Intake.vi"("Effort"=0.0) -> ()  [unwired: 11 in]
          }
        }
      }
      frame "Test" {
      }
      frame "Gear0" {
        n92 = flat-sequence {
          tunnel: w146 -> [w151]
          tunnel: w145 -> [w147]
          frame #0 {
            n93 = To Unsigned Byte Integer(number=w151) -> (unsigned 8bit integer=w150:u8)
            n94 = Wait (ms)(milliseconds to wait=w147) -> ()  [unwired: 1 out]
            n95 = Number To Boolean Array(number=w150) -> (Boolean array=w149:bool[])
            n96 = Index Array(array=w149) -> (element=w148:bool)  [unwired: 1 in]
            n97 = call "Gear.vi"("Gear0?"=w148) -> ()  [unwired: 11 in]
          }
        }
      }
      frame "Gear1" {
        n98 = flat-sequence {
          tunnel: w152 -> [w156]
          frame #0 {
            n99 = To Unsigned Byte Integer(number=w156) -> (unsigned 8bit integer=w155:u8)
            n100 = Number To Boolean Array(number=w155) -> (Boolean array=w154:bool[])
            n101 = Index Array(array=w154) -> (element=w153:bool)  [unwired: 1 in]
            n102 = call "Gear.vi"("Gear1?"=w153) -> ()  [unwired: 11 in]
          }
        }
      }
      frame "Index" {
        n103 = flat-sequence {
          tunnel: w157 -> [w158]
          frame #0 {
            n104 = Wait (ms)(milliseconds to wait=w158) -> ()  [unwired: 1 out]
            n105 = call "Index.vi"("Shoot"=TRUE ("Override?"), "Output"=-1.0) -> ()  [unwired: 10 in]
          }
          frame #1 {
            n106 = call "Index.vi"("Shoot"=FALSE ("Override?"), "Output"=0.0) -> ()  [unwired: 10 in]
          }
        }
      }
      frame "Climb" {
        n107 = flat-sequence {
          tunnel: w164 -> [w166]
          tunnel: w163 -> [w165]
          frame #0 {
            n108 = call "Climb.vi"("Effort"=w166) -> ()  [unwired: 11 in]
            n109 = Wait (ms)(milliseconds to wait=w165) -> ()  [unwired: 1 out]
          }
          frame #1 {
            n110 = call "Climb.vi"("Effort"=0.0) -> ()  [unwired: 11 in]
          }
        }
      }
      frame "Drive Encoder Reset" {
        n111 = while {
          tunnel: w168 -> [w171]
          i -> [w173]
          stop <- w169 stop-if-true
          n112 = Tick Count (ms)() -> (millisecond timer value=w179:u32)
          n113 = Equal?(x=w173, y=0) -> (x = y?=w177:bool)
          n114 = feedback #3(w179) -> (w178:u32)
          n115 = Select(t=w179, s=w177, f=w178) -> (s? t:f=w175:u32)
          n116 = feedback-in #3(w175) -> ()
          n117 = call <vilib>:"WPI_MotorControlRefNum Registry Get.vi"("refnum name"="Drive R1") -> ("error out"=w194:errorcluster, "MotorControlDevRef"=w193:T5)  [unwired: 9 in]
          n118 = call <vilib>:"WPI_MotorControlRefNum Registry Get.vi"("refnum name"="Drive L1") -> ("error out"=w189:errorcluster, "MotorControlDevRef"=w184:T5)  [unwired: 9 in]
          n119 = call <vilib>:"WPI_MotorControlRefNum Registry Get.vi"("refnum name"="Drive R1") -> ("error out"=w186:errorcluster, "MotorControlDevRef"=w185:T5)  [unwired: 9 in]
          n120 = Subtract(x=w179, y=w175) -> (x-y=w172:u32)
          n121 = call <vilib>:"WPI_MotorControlRefNum Registry Get.vi"("refnum name"="Drive L1") -> ("error out"=w196:errorcluster, "MotorControlDevRef"=w197:T5)  [unwired: 9 in]
          n122 = call <vilib>:"WPI_CANTalonSRX_SetSensorPosition.vi"("error in (no error)"=w194, "New Sensor Position"=0.0, "CAN Talon SRX Ref"=w193) -> ()  [unwired: 7 in, 2 out]
          n123 = call <vilib>:"WPI_CANTalonSRX_GetStatus.vi"("error in (no error)"=w189, "CAN Talon SRX Ref"=w184) -> ("Talon SRX Status"=w187:T9)  [unwired: 7 in, 2 out]
          n124 = call <vilib>:"WPI_CANTalonSRX_GetStatus.vi"("error in (no error)"=w186, "CAN Talon SRX Ref"=w185) -> ("Talon SRX Status"=w188:T9)  [unwired: 7 in, 2 out]
          n125 = call <vilib>:"WPI_CANTalonSRX_SetSensorPosition.vi"("error in (no error)"=w196, "New Sensor Position"=0.0, "CAN Talon SRX Ref"=w197) -> ()  [unwired: 7 in, 2 out]
          n126 = Unbundle By Name(w187) -> ("Encoder Position"=w182:dbl)
          n127 = Unbundle By Name(w188) -> ("Encoder Position"=w183:dbl)
          n128 = Greater?(x=w172, y=w171) -> (0:w170:bool)
          n129 = Equal To 0?(x=w182) -> (x = 0?=w181:bool)
          n130 = Equal To 0?(x=w183) -> (x = 0?=w180:bool)
          n131 = And(x=w181, y=w180) -> (x .and. y?=w174:bool)
          n132 = And(x=w170, y=w174) -> (x .and. y?=w169:bool)
        }
      }
      frame "Gyro Reset" {
        n133 = while {
          stop <- w200 stop-if-true
          w203 = 0.3
          n134 = global read "Global 2.vi" "Gyro"() -> (w201:dbl)
          n135 = Negate(x=w203) -> (-x=w202:dbl)
          n136 = call <vilib>:"WPI_GyroRefNum Registry Get.vi"("refnum name"="Gyro") -> ("error out"=w205:errorcluster, "GyroDevRef"=w206:T10)  [unwired: 9 in]
          n137 = call <vilib>:"WPI_GyroReset.vi"("error in"=w205, "GyroDevRef"=w206) -> ()  [unwired: 8 in, 2 out]
          n138 = In Range and Coerce(upper limit=w203, x=w201, lower limit=w202) -> (In Range?=w200:bool)  [unwired: 1 out]
        }
      }
    }
  }
